vi "Initialize Hardware.vi"(8 "error in":errorcluster) -> (0 "error out":errorcluster)   [LabVIEW 2015]
uses:
  CAN Communication/PAS/Typedefs/Valves.ctl
  CAN Communication/PAS/PAS.lvclass
panel:
  in  "Valves":T1=17 items=["GV1"=17, "GV2"=18, "GV3"=19, "GV4"=20]
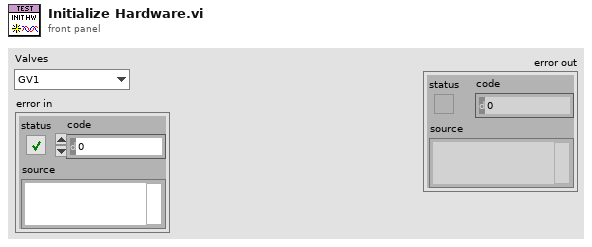
[diagram p1: front panel]
types:
  T1 = typedef "PAS.lvclass/Valves.ctl" = u16
  T2 = typedef "LVStringsAndValuesArrayTypeDef_U16.ctl" = cluster{"String":string, "Value":u16}[]
  T3 = typedef "PAS.lvclass/Session Handle.ctl" = refnum<data-value>
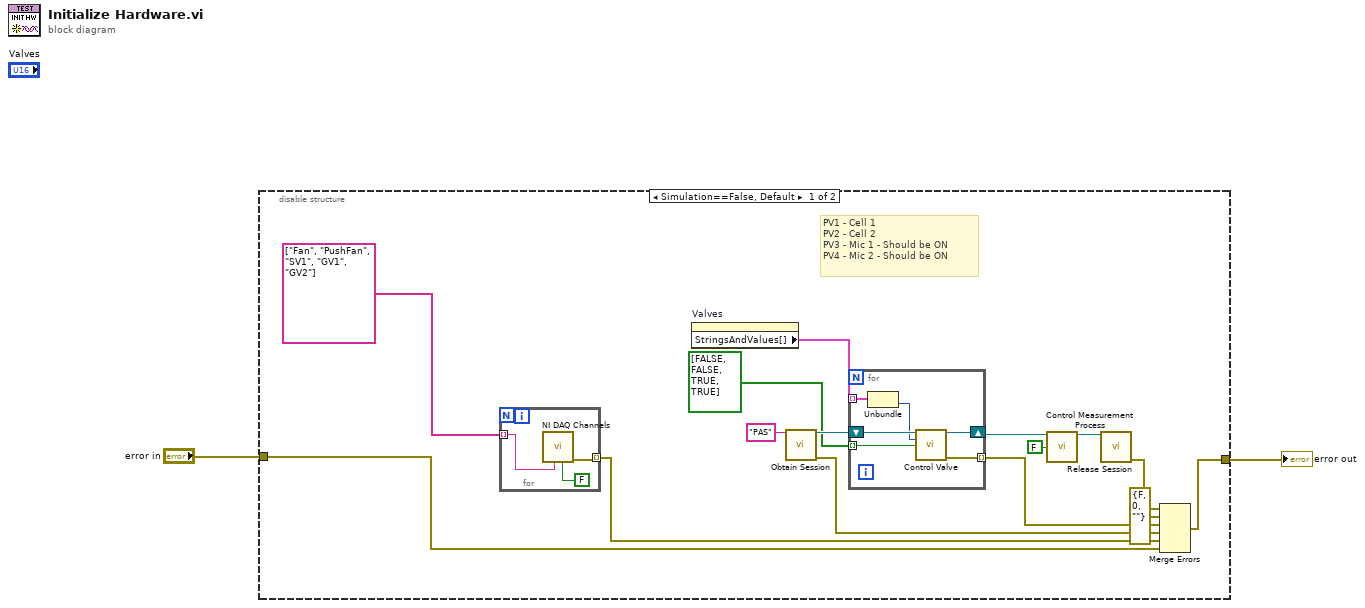
[diagram p0: block diagram]
diagram:
  n1 = disable-structure shown="Simulation==False, Default" {
    disable-tunnel: "error in" -> [w7 w27]
    disable-tunnel: [w12 w27] -> w1
    frame condition #0 (active) {
      # "PV1 - Cell 1\nPV2 - Cell 2\nPV3 - Mic 1 - Should be ON\nPV4 - Mic 2 - Should be ON"
      n2 = for {
        tunnel: [w20] -> w8 mode=indexing
        tunnel: string[] ["Fan", "PushFan", "SV1", "GV1", "GV2"] -> [w19] mode=indexing
        n3 = call "NI DAQ Channels.vi"("Control"=FALSE, "Channel"=w19) -> ("error out"=w20:errorcluster)  [unwired: 8 in, 1 out]
      }
      n4 = property on="Valves" class="Ring (strict)"() -> ("StringsAndValues[]"=w15:T2)  [unwired: 2 in, 2 out]
      n5 = call "Obtain Session.vi"("Session  Name ()"="PAS") -> ("Session Handle"=w16:T3, "error out"=w9:errorcluster)  [unwired: 13 in]
      n6 = for {
        shift-right: [w25] -> w14
        shift-left: w16 -> [w26]
        tunnel: w15 -> [w24] mode=indexing
        tunnel: [w22] -> w10 mode=indexing
        tunnel: bool[] [FALSE, FALSE, TRUE, TRUE] -> [w21] mode=indexing
        n7 = Unbundle(w24) -> ("Value"=w23:u16)  [unwired: 1 out]
        n8 = call "Control Valve.vi"("Session Handle in"=w26, "Valves"=w23, "Energize?"=w21) -> ("Session Handle out"=w25:T3, "error out"=w22:errorcluster)  [unwired: 9 in, 2 out]
      }
      n9 = call "Control Measurement Process.vi"("Session Handle in"=w14, "Start?"=FALSE) -> ("Session Handle out"=w13:T3)  [unwired: 10 in, 3 out]
      n10 = call "Release Session.vi"("Session Handle"=w13) -> ("error out"=w11:errorcluster)  [unwired: 14 in]
      n11 = Merge Errors(w11, errorcluster {"status"=FALSE, "code"=0, "source"=""} ("error in"), w10, w9, w8, w7) -> (w12:errorcluster)
    }
    frame condition #1 {
    }
  }
  "error out" <- w1
